vi "3B_Chrg_Discharge.vi"() -> ()   [LabVIEW 2020]
panel:
  in  "Capacity (Ah)":dbl format="%#.6g"
  in  "Starting Cycle":i32
  in  "Wait time (s)":dbl
  in  "p task error in":errorcluster
  in  "Parallel Task in":refnum<k21>
  in  "C rate Setpoint":dbl format="%#.6g"
  in  "NHR error in":errorcluster caption="error in (no error)"
  in  "NHR VISA":refnum<visa-resource-name>
  in  "task error in":errorcluster
  in  "Relay Task":refnum<k21>
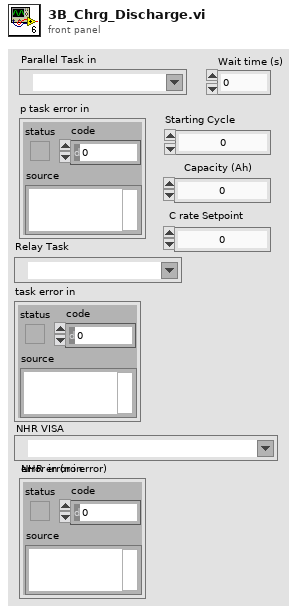
[diagram p1: front panel]
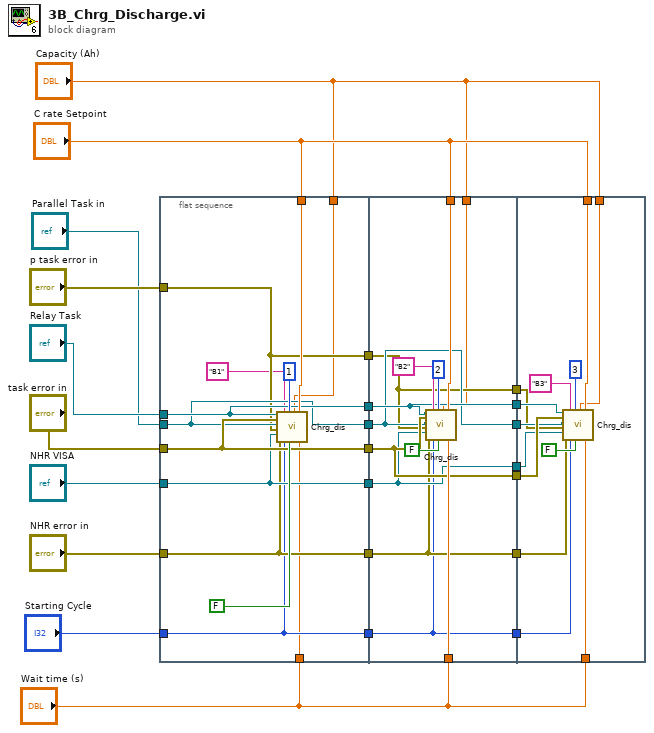
[diagram p0: block diagram]
diagram:
  n1 = flat-sequence {
    tunnel: "Relay Task" -> [w34]
    tunnel: "task error in" -> [w33]
    tunnel: "NHR VISA" -> [w30]
    tunnel: "NHR error in" -> [w29]
    tunnel: "p task error in" -> [w31]
    tunnel: "Parallel Task in" -> [w32]
    tunnel: "C rate Setpoint" -> [w36]
    tunnel: "Wait time (s)" -> [w26]
    tunnel: "Starting Cycle" -> [w28]
    tunnel: [w34] -> w17
    tunnel: [w33] -> w16
    tunnel: [w32] -> w15
    tunnel: [w31] -> w14
    tunnel: [w30] -> w13
    tunnel: [w29] -> w12
    tunnel: [w28] -> w11
    tunnel: "Capacity (Ah)" -> [w25]
    tunnel: w17 -> [w45]
    tunnel: w16 -> [w44]
    tunnel: w15 -> [w43]
    tunnel: w14 -> [w42]
    tunnel: w13 -> [w41]
    tunnel: w12 -> [w40]
    tunnel: w11 -> [w39]
    tunnel: "C rate Setpoint" -> [w47]
    tunnel: "Wait time (s)" -> [w46]
    tunnel: [w45] -> w10
    tunnel: [w44] -> w9
    tunnel: [w43] -> w8
    tunnel: [w42] -> w7
    tunnel: [w41] -> w6
    tunnel: [w40] -> w5
    tunnel: [w39] -> w4
    tunnel: "Capacity (Ah)" -> [w38]
    tunnel: w10 -> [w60]
    tunnel: w9 -> [w59]
    tunnel: w8 -> [w58]
    tunnel: w7 -> [w57]
    tunnel: w6 -> [w56]
    tunnel: w5 -> [w55]
    tunnel: w4 -> [w54]
    tunnel: "Wait time (s)" -> [w53]
    tunnel: "C rate Setpoint" -> [w52]
    tunnel: "Capacity (Ah)" -> [w51]
    frame #0 {
      n2 = call "Chrg_dis.vi"("Relay Task"=w34, "task error in"=w33, "Parallel Task in"=w32, "P task error in"=w31, "NHR VISA"=w30, "NHR error in"=w29, "Batteryname"="B1", "Starting Cycle"=w28, "Battery Select"=1, "In for loop?"=FALSE, "Capacity (Ah)"=w25, "C rate Setpoint"=w36, "Wait time (s)"=w26) -> ()  [unwired: 7 in]
    }
    frame #1 {
      n3 = call "Chrg_dis.vi"("Relay Task"=w45, "task error in"=w44, "Parallel Task in"=w43, "P task error in"=w42, "NHR VISA"=w41, "NHR error in"=w40, "Batteryname"="B2", "Starting Cycle"=w39, "Battery Select"=2, "In for loop?"=FALSE, "Capacity (Ah)"=w38, "C rate Setpoint"=w47, "Wait time (s)"=w46) -> ()  [unwired: 7 in]
    }
    frame #2 {
      n4 = call "Chrg_dis.vi"("Relay Task"=w60, "task error in"=w59, "Parallel Task in"=w58, "P task error in"=w57, "NHR VISA"=w56, "NHR error in"=w55, "Batteryname"="B3", "Starting Cycle"=w54, "Battery Select"=3, "In for loop?"=FALSE, "Capacity (Ah)"=w51, "C rate Setpoint"=w52, "Wait time (s)"=w53) -> ()  [unwired: 7 in]
    }
  }
